vi "Extended Actor Template-Core_Initialize.vi"(0 "Initialization Sequence":string, 5 "FTW Actor Instance Configuration":string, 11 "error in (no error)":errorcluster) -> (4 "Actor Template-Core out":refnum<class "Extended Actor Template-Core.lvclass">, 6 "Event Refnums":T1, 10 "Refresh Period":dbl, 15 "error out":errorcluster)   [LabVIEW 2015, in "Extended Actor Template-Core.lvclass"]
uses:
  Extended Actor Template-Core.lvclass
  source/actor/Message/Request/FTW-Message-IncomingRequest.lvclass
  source/actor/Message/Base/FTW-Message.lvclass
  Extended Actor Template-Core.lvclass/Extended Actor Template-Core.ctl
  source/JSON/core/FTW-JSON-Core-EncodingFlags.vi
  source/JSON/FTW-JSON-Parse.vi
  source/Reflection/FTW-Reflection-Type.vi
  source/CodeGen/JSON Deserialize/FTW-JSON-Core-GetFlattenedValue.vi
  source/CodeGen/JSON Deserialize/FTW-JSON-Deserialize.xnode
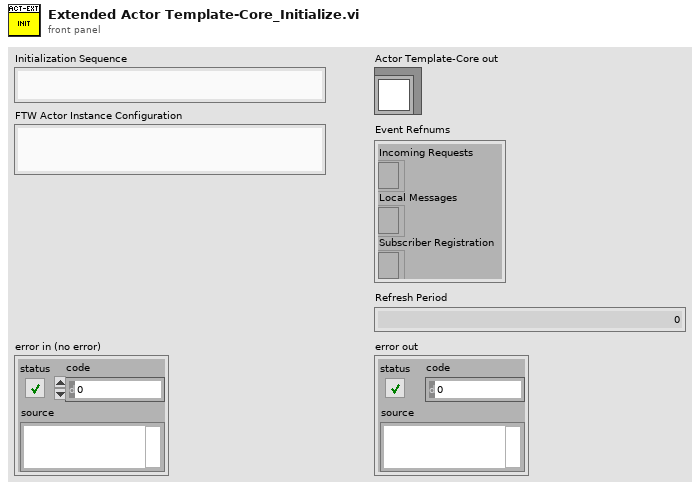
[diagram p1: front panel]
types:
  T1 = cluster{"Incoming Requests":refnum<event-registration>, "Local Messages":refnum<event-registration>, "Subscriber Registration":refnum<event-registration>}
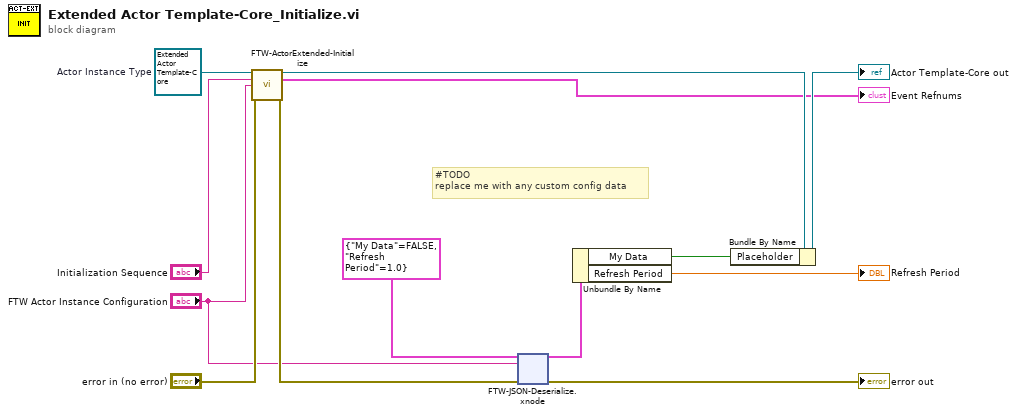
[diagram p0: block diagram]
diagram:
  w1 = refnum<class "Extended Actor Template-Core.lvclass"> refnum  # Actor Instance Type
  # "#TODO\nreplace me with any custom config data"
  n1 = call-dynamic "FTW-ActorExtended-Initialize.vi"("FTW Actor Instance Type"=w1, "Initialization Job Sequence"="Initialization Sequence", "Actor Instance Configuration"="FTW Actor Instance Configuration", "error in"="error in (no error)") -> ("FTW Actor Instance"=w8:refnum<class "Extended Actor Template-Core.lvclass">, "Event Refnums"=→"Event Refnums":T1, "error out"=w6:errorcluster)  [unwired: 9 in]
  n2 = xnode "FTW-JSON-Deserialize.xnode"("Type and Defaults"=cluster{"My Data":bool, "Refresh Period":dbl} {"My Data"=FALSE, "Refresh Period"=1.0}, "JSON String"="FTW Actor Instance Configuration", "error in"=w6) -> ("Values"=w10:cluster{"My Data":bool, "Refresh Period":dbl}, "error out"=→"error out":errorcluster)
  n3 = Unbundle By Name(w10) -> ("My Data"=w9:bool, "Refresh Period"=→"Refresh Period":dbl)
  n4 = Bundle By Name(cluster=w8, "Placeholder"=w9) -> (→"Actor Template-Core out":refnum<class "Extended Actor Template-Core.lvclass">)
